vi "DAQmx Create Channel (AI-Acceleration-Charge).vi"(0 "task in":refnum<k21>, 1 "maximum value":dbl=5.0 format="%0.5f", 2 "minimum value":dbl=-5.0 format="%0.5f", 3 "input terminal configuration":i32(ring)=-1 items=["Default"=-1, "RSE"=10083, "NRSE"=10078, "Differential"=10106, "Pseudodifferential"=12529], 5 "physical channels":tag, 7 "name to assign":string, 9 "units":i32(ring)=10186 items=["g"=10186, "m/s^2"=12470, "in/s^2"=12471, "From Custom Scale"=10065], 11 "error in":errorcluster, 12 "custom scale name":tag, 13 "sensitivity":dbl=100.0, 14 "sensitivity units":i32(ring)=16099 items=["pCoulomb/g"=16099, "pCoulomb/(m/s^2)"=16100, "pCoulomb/(in/s^2)"=16101]) -> (4 "task out":refnum<k21>, 15 "error out":errorcluster)   [LabVIEW 2013]
doc: "Creates channel(s) that use a charge-based sensor to measure acceleration."
uses:
  nilvaiu.dll
panel:
  # "input limits"
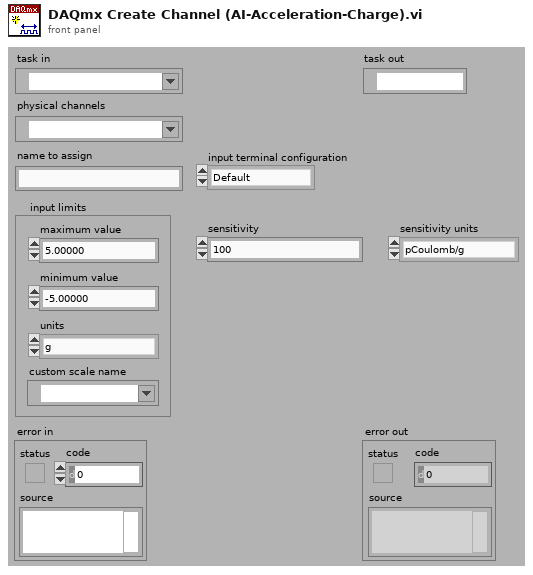
[diagram p1: front panel]
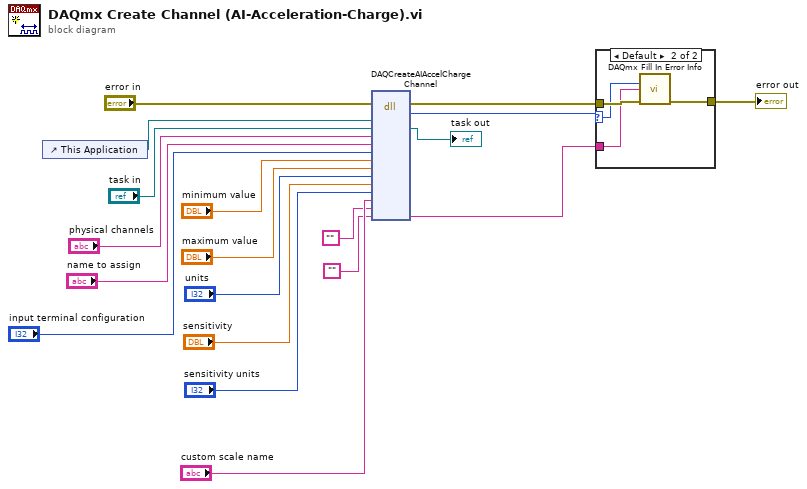
[diagram p0: block diagram]
diagram:
  n1 = control-ref of="This Application"() -> (w18:refnum<vi>)
  n2 = dll-call lib="nilvaiu.*" fn="DAQCreateAIAccelChargeChannel"(error in="error in", "lvAppReference"=w18, "taskID"="task in", "physical channel name"="physical channels", "virtual channel name"="name to assign", "input terminal configuration"="input terminal configuration", "minimum value"="minimum value", "maximum value"="maximum value", "units"="units", "sensitivity"="sensitivity", "sensitivity units"="sensitivity units", "customScale"="custom scale name", "channelNamesOut"="", "extendedErrorIndo"="") -> (error out=w6:errorcluster, "return type"=w4:i32, "taskID"=→"task out":refnum<k21>, "extendedErrorIndo"=w5:string)  [unwired: 13 in, 1 out]
  n3 = case shown="Default" w4 {
    selector: w4 -> [_ w22]
    tunnel: w6 -> [w20 w24]
    tunnel: [w20 w23] -> w7
    tunnel: w5 -> [_ w21]
    frame 0 {
    }
    frame Default {
      n4 = call "DAQmx Fill In Error Info.vi"("status code"=w22, "extended error info"=w21, "error in"=w24) -> ("error out"=w23:errorcluster)  [unwired: 1 in, 11 out]
    }
  }
  "error out" <- w7
